vi "PPMU_Meas.vi"(7 "HDSIO_PPMU_Settings":T1={"voltage level"=1.8, "current range"=0.0, "aperture time (4E-6 s)"=4e-06} {"current range" format="%#_6p"}, 8 "Error In":errorcluster, 10 "channel list":string="0", 11 "HSDIO Sessions":T2) -> (0 "Error Out":errorcluster, 1 "current measurements":dbl[](array[numeric]), 2 "voltage measurements":dbl[](array[numeric]), 3 "HSDIO Sessions":T2)   [LabVIEW 2013]
uses:
  <instrlib>/niHSDIO/niHSDIO.llb/niHSDIO_ctl stPMU Disable Return State.ctl
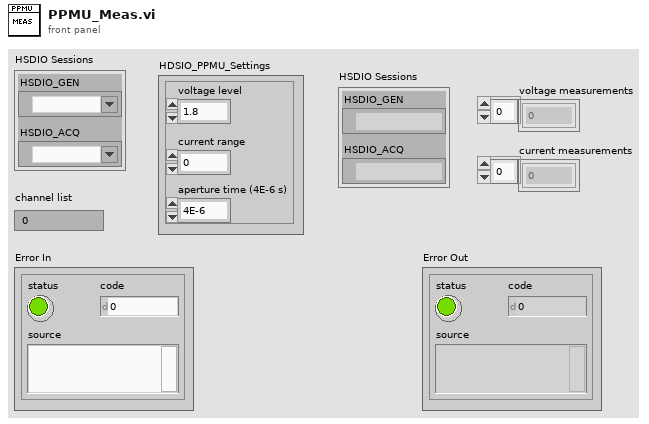
[diagram p1: front panel]
types:
  T1 = cluster{"voltage level":dbl, "current range":dbl, "aperture time (4E-6 s)":dbl}
  T2 = cluster{"HSDIO_ACQ":refnum<k15>, "HSDIO_GEN":refnum<k15>}
  T3 = typedef "niHSDIO_ctl stPMU Disable Return State.ctl" = u32
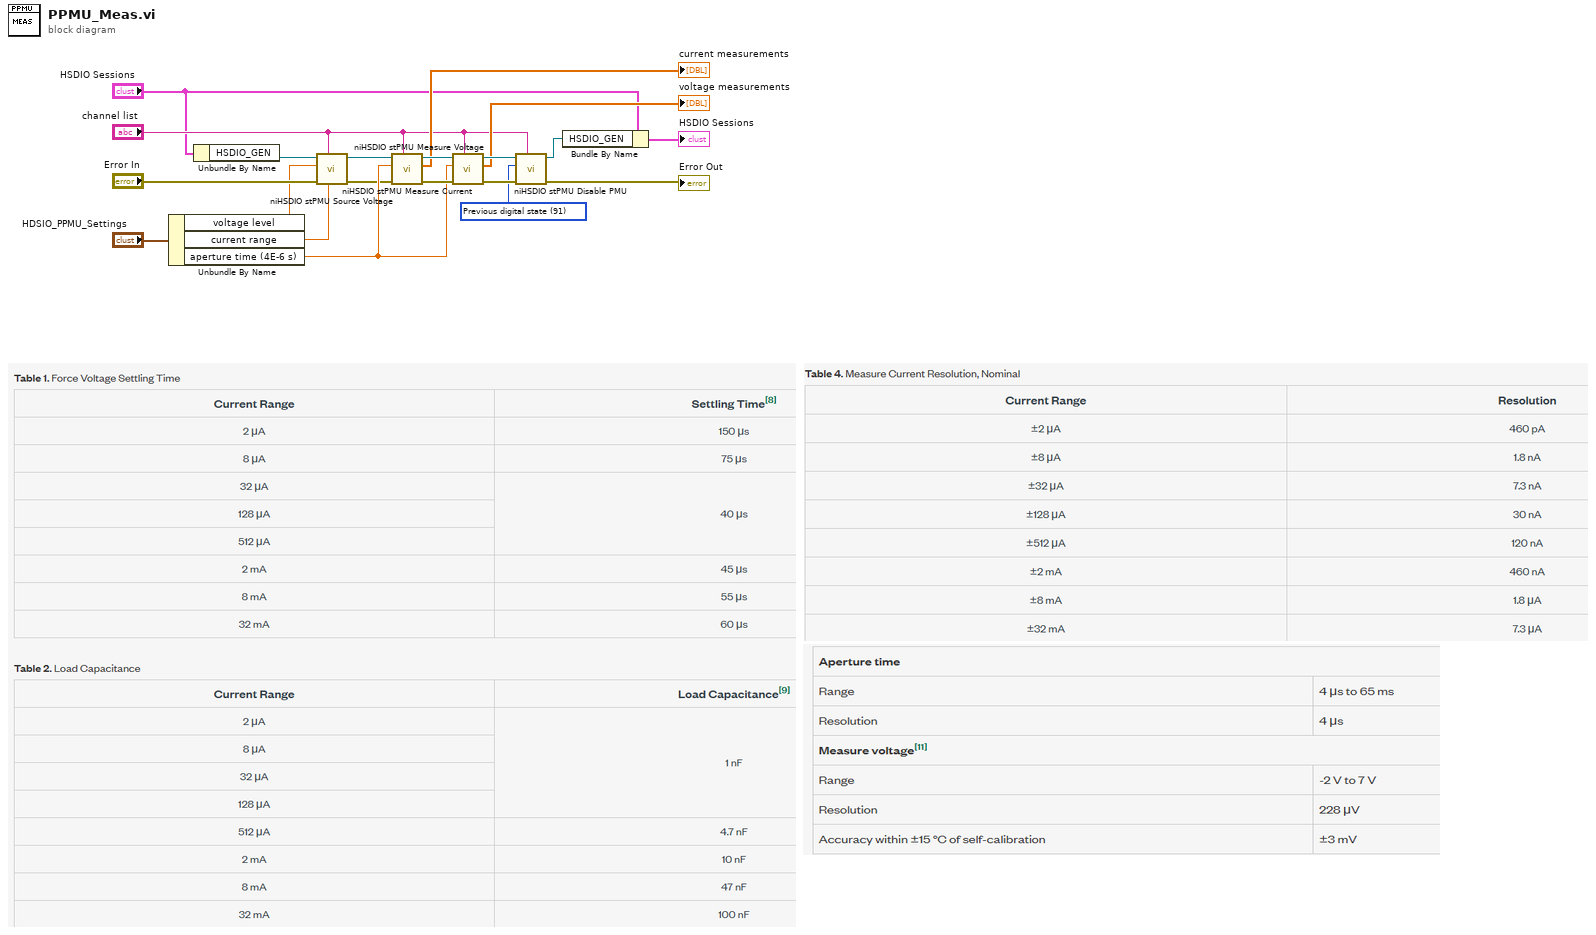
[diagram p0: block diagram]
diagram:
  w12 = T3 91 items=["Tristate"=90, "Previous digital state"=91] ("return state (tristate)")
  n1 = Unbundle By Name("HDSIO_PPMU_Settings") -> ("voltage level"=w6:dbl, "current range"=w5:dbl, "aperture time (4E-6 s)"=w4:dbl)
  n2 = Unbundle By Name("HSDIO Sessions") -> ("HSDIO_GEN"=w15:refnum<k15>)
  n3 = call <instrlib>:"niHSDIO stPMU Source Voltage.vi"("current range"=w5, "channel list"="channel list", "error in (no error)"="Error In", "voltage level"=w6, "instrument handle"=w15) -> ("error out"=w2:errorcluster, "instrument handle out"=w1:refnum<k15>)  [unwired: 5 in]
  n4 = call <instrlib>:"niHSDIO stPMU Measure Current.vi"("channel list"="channel list", "error in (no error)"=w2, "aperture time (4E-6 s)"=w4, "instrument handle"=w1) -> ("error out"=w20:errorcluster, "current measurements"=→"current measurements":dbl[], "instrument handle out"=w17:refnum<k15>)  [unwired: 5 in]
  n5 = call <instrlib>:"niHSDIO stPMU Measure Voltage.vi"("channel list"="channel list", "error in (no error)"=w20, "aperture time (4E-6 s)"=w4, "instrument handle"=w17) -> ("error out"=w19:errorcluster, "voltage measurements"=→"voltage measurements":dbl[], "instrument handle out"=w16:refnum<k15>)  [unwired: 5 in]
  n6 = call <instrlib>:"niHSDIO stPMU Disable PMU.vi"("channel list"="channel list", "error in (no error)"=w19, "return state (tristate)"=w12, "instrument handle"=w16) -> ("error out"=→"Error Out":errorcluster, "instrument handle out"=w9:refnum<k15>)  [unwired: 6 in]
  n7 = Bundle By Name(cluster="HSDIO Sessions", "HSDIO_GEN"=w9) -> (→"HSDIO Sessions":T2)
